vi "F Dwf Analog Out Node Phase Info.vi"(6 "pdegreeMax":dbl, 7 "pdegreeMin":dbl, 8 "error in (no error)":errorcluster, 9 "node":i32, 10 "idxChannel":i32, 11 "hdwf":i32) -> (0 "error out":errorcluster, 3 "function return":i32, 4 "pdegreeMax out":dbl, 5 "pdegreeMin out":dbl)   [LabVIEW 2021, in "Olasdwf.lvlib"]
doc: "DWFAPI int FDwfAnalogOutNodePhaseInfo(HDWF hdwf, int idxChannel, AnalogOutNode node, double *pdegreeMin, double *pdegreeMax);"
uses:
  Olasdwf.lvlib
  Windows/System32/dwf.dll
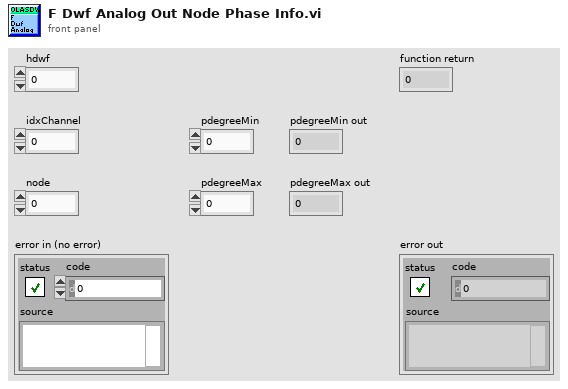
[diagram p1: front panel]
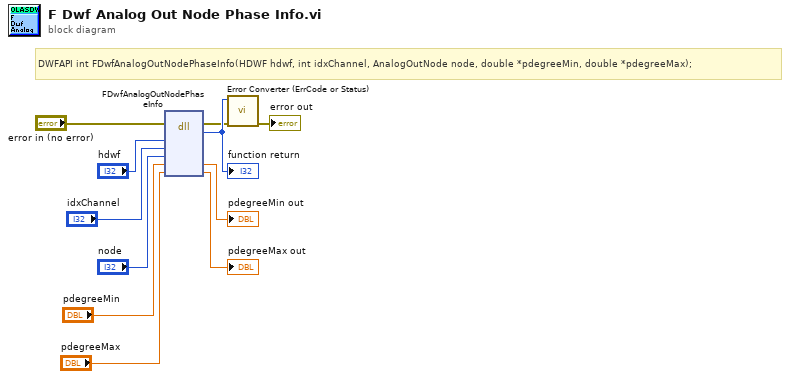
[diagram p0: block diagram]
diagram:
  # "DWFAPI int FDwfAnalogOutNodePhaseInfo(HDWF hdwf, int idxChannel, AnalogOutNode node, double *pdegreeMin, double *pdegreeMax);"
  n1 = dll-call lib="/Windows/System32/dwf.*" fn="FDwfAnalogOutNodePhaseInfo"(error in="error in (no error)", "hdwf"="hdwf", "idxChannel"="idxChannel", "node"="node", "pdegreeMin"="pdegreeMin", "pdegreeMax"="pdegreeMax") -> (error out=w2:errorcluster, w11:i32, "pdegreeMin"=→"pdegreeMin out":dbl, "pdegreeMax"=→"pdegreeMax out":dbl)  [unwired: 5 in, 1 out]
  "function return" <- w11
  n2 = call "Error Converter (ErrCode or Status).vi"("error in (no error)"=w2, "error code"=w11) -> ("error out"=→"error out":errorcluster)  [unwired: 9 in]
